vi "GV Nmax lines.vi"() -> ()   [LabVIEW 2017]
panel:
  in  "Nmax lines":u16
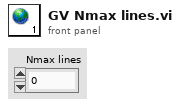
[diagram p1: front panel]
diagram:
